vi "Doc_Builder_Save_Close_Report.vi"(10 "appended path":path, 11 "NI_report in":refnum<class "NI_report.lvclass">) -> (0 "error out":errorcluster)   [LabVIEW 2019]
uses:
  <vilib>/Utility/NIReport.llb/NI_report.lvclass
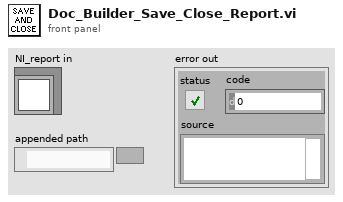
[diagram p1: front panel]
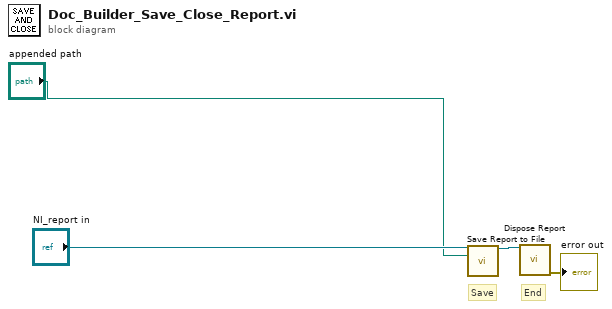
[diagram p0: block diagram]
diagram:
  # "End"
  # "Save"
  n1 = call-dynamic "Save Report to File.vi"("report in"="NI_report in", "report file path"="appended path") -> ("report out"=w1:refnum<class "NI_report.lvclass">)  [unwired: 12 in, 1 out]
  n2 = call-dynamic "Dispose Report.vi"("report in"=w1) -> ("error out"=→"error out":errorcluster)  [unwired: 14 in]
